vi "Apply.vi"(8 "error in":errorcluster, 11 "DIO DO PWM DI Meas Freq CFG in":refnum<class "DIO DO PWM DI Meas Freq CFG.lvclass">) -> (0 "error out":errorcluster, 3 "DIO DO PWM DI Meas Freq CFG out":refnum<class "DIO DO PWM DI Meas Freq CFG.lvclass">)   [LabVIEW 2023, in "DIO DO PWM DI Meas Freq CFG.lvclass"]
uses:
  DIO DO PWM DI Meas Freq CFG.lvclass
  DIO DO PWM DI Meas Freq CFG.lvclass/DIO DO PWM DI Meas Freq CFG.ctl
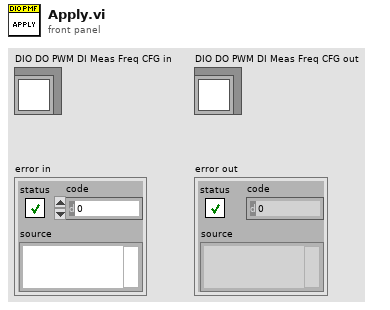
[diagram p1: front panel]
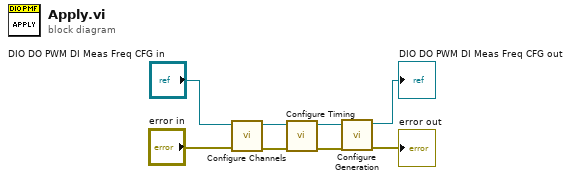
[diagram p0: block diagram]
diagram:
  n1 = call-dynamic "Configure Channels.vi"("error in"="error in", "DIO DO PWM DI Meas Freq CFG in"="DIO DO PWM DI Meas Freq CFG in") -> ("error out"=w5:errorcluster, "DIO DO PWM DI Meas Freq CFG out"=w6:refnum<class "DIO DO PWM DI Meas Freq CFG.lvclass">)  [unwired: 8 in]
  n2 = call-dynamic "Configure Timing.vi"("error in"=w5, "DAQmx Base CFG in"=w6) -> ("error out"=w4:errorcluster, "DAQmx Base CFG out"=w3:refnum<class "DIO DO PWM DI Meas Freq CFG.lvclass">)  [unwired: 8 in]
  n3 = call-dynamic "Configure Generation.vi"("error in"=w4, "DIO DO PWM DI Meas Freq CFG in"=w3) -> ("error out"=→"error out":errorcluster, "DIO DO PWM DI Meas Freq CFG out"=→"DIO DO PWM DI Meas Freq CFG out":refnum<class "DIO DO PWM DI Meas Freq CFG.lvclass">)  [unwired: 8 in]
